vi "颗粒滤波3 filter.vi"() -> ()   [LabVIEW 2018]
uses:
  <vilib>/vision/NI_Vision_Development_Module.lvlib
panel:
  in  "Selection Values":T2(array[cluster])=[{"Measurement Parameter"=39, "Range Lower Value"=5.0, "Range Upper Value"=10000000.0, "Range"=FALSE, "Measurement Type"=FALSE}] {"Measurement Parameter" items=["Center of Mass X", "Center of Mass Y", "First Pixel X", "First Pixel Y", "Bounding Rect Left", "Bounding Rect Top", "Bounding Rect Right", "Bounding Rect Bottom", "Max Feret Diameter Start X", "Max Feret Diameter Start Y", "Max Feret Diameter End X", "Max Feret Diameter End Y", "Max Horiz. Segment Length Left", "Max Horiz. Segment Length Right", "Max Horiz. Segment Length Row", "-", "Bounding Rect Width", "Bounding Rect Height", "Bounding Rect Diagonal", "Perimeter", "Convex Hull Perimeter", "Holes' Perimeter", "Max Feret Diameter", "Equivalent Ellipse Major Axis", "Equivalent Ellipse Minor Axis", "Equivalent Ellipse Minor Axis (Feret)", "Equivalent Rect Long Side", "Equivalent Rect Short Side", "Equivalent Rect Diagonal", "Equivalent Rect Short Side (Feret)", "Average Horiz. Segment Length", "Average Vert. Segment Length", "Hydraulic Radius", "Waddel Disk Diameter", "-", "Area", "Holes' Area", "Particle & Holes' Area", "Convex Hull Area", "Image Area", "-", "Number of Holes", "Number of Horiz. Segments", "Number of Vert. Segments", "-", "Orientation", "Max Feret Diameter Orientation", "-", "% Area/Image Area", "% Area/(Particle & Holes' Area)", "Ratio of Equivalent Ellipse Axes", "Ratio of Equivalent Rect Sides", "-", "Elongation Factor", "Compactness Factor", "Heywood Circularity Factor", "Type Factor", "-", "Sum X", "Sum Y", "Sum XX", "Sum XY", "Sum YY", "Sum XXX", "Sum XXY", "Sum XYY", "Sum YYY", "-", "Moment of Inertia XX", "Moment of Inertia XY", "Moment of Inertia YY", "Moment of Inertia XXX", "Moment of Inertia XXY", "Moment of Inertia XYY", "Moment of Inertia YYY", "Norm. Moment of Inertia XX", "Norm. Moment of Inertia XY", "Norm. Moment of Inertia YY", "Norm. Moment of Inertia XXX", "Norm. Moment of Inertia XXY", "Norm. Moment of Inertia XYY", "Norm. Moment of Inertia YYY", "Hu Moment 1", "Hu Moment 2", "Hu Moment 3", "Hu Moment 4", "Hu Moment 5", "Hu Moment 6", "Hu Moment 7"]}
  in  "Tab Control":T3(tab)
  out "Original":T4(plugin-control) caption="Original Image"
  out "Threshold":T4(plugin-control) caption="Threshold Image"
  out "Fill Hole and Reject Border":T4(plugin-control) caption="Reject Border and Fill Holes"
  out "Filter and Overlay Area":T4(plugin-control) caption="Filter Out Non Circles and Overlay Particle Area"
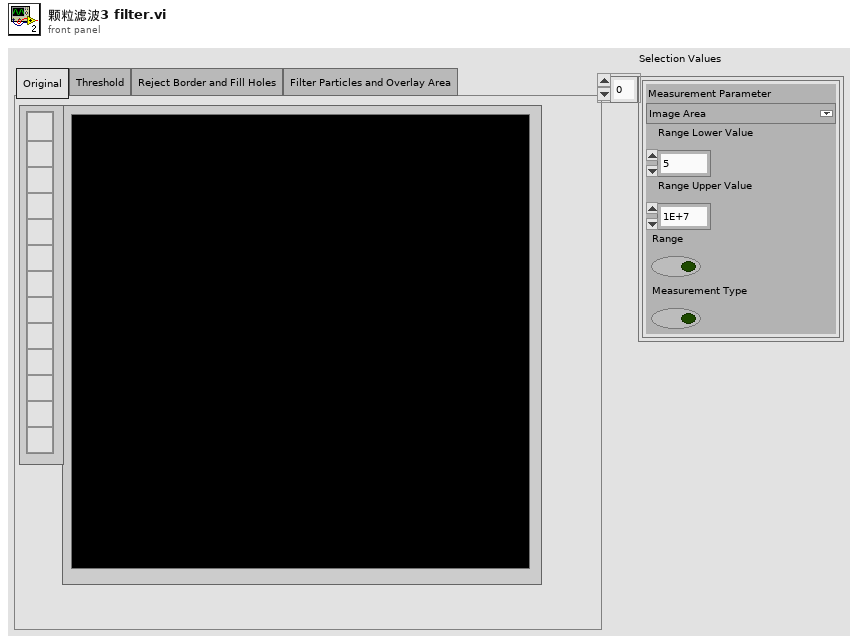
[diagram p1: front panel]
types:
  T1 = typedef "Particle Parameters" = i32
  T2 = cluster{"Measurement Parameter":T1, "Range Lower Value":dbl, "Range Upper Value":dbl, "Range":bool, "Measurement Type":bool}[]
  T3 = enum32{"Original", "Threshold", "Reject Border and Fill Holes", "Filter Particles and Overlay Area"}
  T4 = typedef "IMAQ Image.ctl" = refnum<image>
  T5 = typedef "Image Type" = u32
  T6 = cluster{"Desired Font (Application)":enum16{"User-specified Font", "Application Font", "System Font", "Dialog Font"}, "[User-specified Font]":cluster{"Font Name":string, "Size":i16, "Strikeout?":bool, "Italic?":bool, "Underline?":bool, "Outline?":bool, "Shadow?":bool, "Bold?":bool, "Rotation Angle":dbl}, "Horizontal Alignment":i16, "Vertical Alignment":i16}
  T7 = cluster{"Particle Measurements (Pixels)[0]":dbl, "Particle Measurements (Pixels)[1]":dbl, "Particle Measurements (Pixels)[2]":dbl}
  T8 = cluster{"Particle Measurements (Pixels)[0]":dbl, "Particle Measurements (Pixels)[1]":dbl}
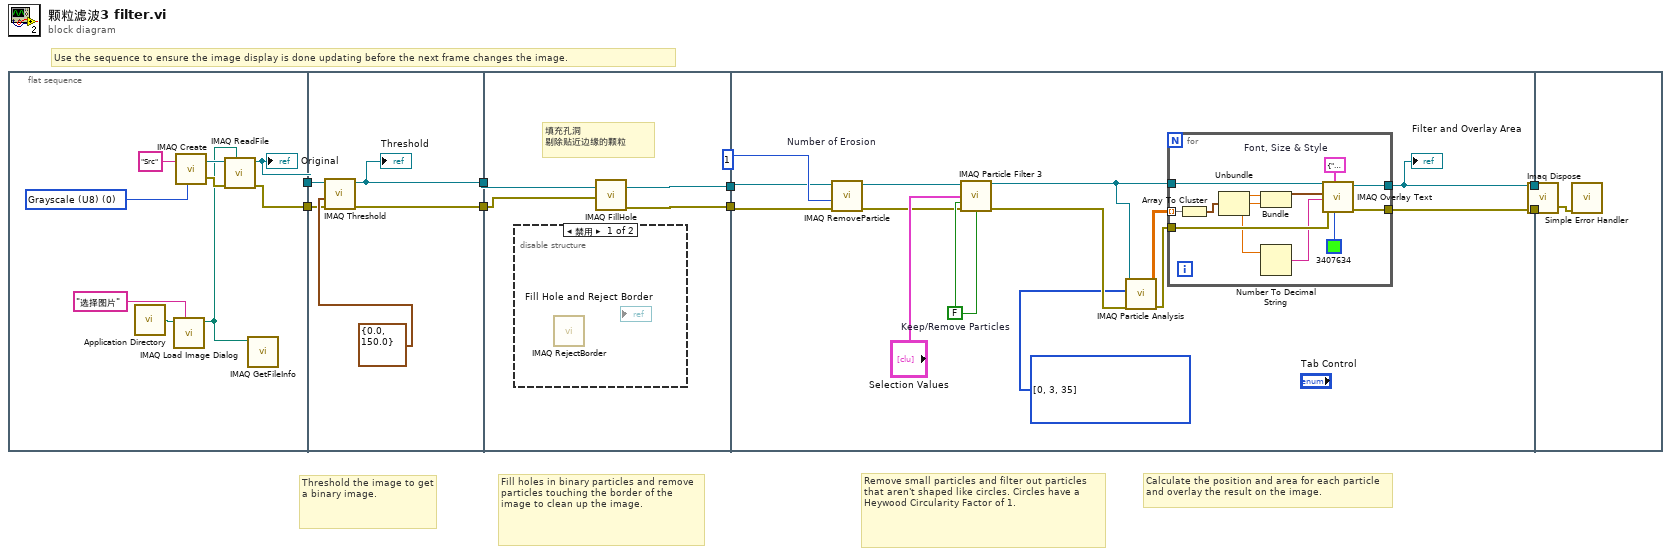
[diagram p0: block diagram]
diagram:
  # "Use the sequence to ensure the image display is done updating before the next frame changes the image."
  # "Calculate the position and area for each particle and overlay the result on the image."
  # "Remove small particles and filter out particles that aren't shaped like circles. Circles have a Heywood Circularity Factor of 1."
  # "Fill holes in binary particles and remove particles touching the border of the image to clean up the image."
  # "Threshold the image to get a binary image."
  n1 = flat-sequence {
    tunnel: [w11] -> w8
    tunnel: [w10] -> w7
    tunnel: [w20] -> w6
    tunnel: [w21] -> w5
    tunnel: w8 -> [w19]
    tunnel: w7 -> [w18]
    tunnel: w6 -> [w26]
    tunnel: w5 -> [w25]
    tunnel: [w24] -> w3
    tunnel: [w23] -> w4
    tunnel: w4 -> [w30]
    tunnel: w3 -> [w29]
    tunnel: [w36] -> w2
    tunnel: [w28] -> w1
    tunnel: w2 -> [w55]
    tunnel: w1 -> [w56]
    frame #0 {
      w12 = T5 0 items=["Grayscale (U8)", "Grayscale (I16)", "Grayscale (SGL)", "Complex (CSG)", "RGB (U32)", "HSL (U32)", "RGB (U64)", "Grayscale (U16)"] ("Image Type")
      n2 = call <vilib>:"Application Directory.vi"() -> ("Application Directory"=w13:path)
      n3 = call "IMAQ Load Image Dialog"("Prompt"="选择图片" ("prompt"), "Start Path"=w13) -> ("Path"=w9:path)  [unwired: 7 in, 2 out]
      n4 = call "IMAQ Create"("Image Name"="Src", "Image Type"=w12) -> ("New Image"=w16:T4, "error out"=w15:errorcluster)  [unwired: 3 in]
      n5 = call "IMAQ ReadFile"("File Path"=w9, "error in (no error)"=w15, "Image"=w16) -> ("error out"=w10:errorcluster, "Image Out"=w11:T4)  [unwired: 4 in, 3 out]
      "Original" <- w11
      n6 = call "IMAQ GetFileInfo"("File Path"=w9) -> ()  [unwired: 4 in, 7 out]
    }
    frame #1 {
      n7 = call "IMAQ Threshold"("error in (no error)"=w18, "Range"=cluster{"Lower value":sgl, "Upper value":sgl} {"Lower value"=0.0, "Upper value"=150.0}, "Image Src"=w19) -> ("error out"=w21:errorcluster, "Image Dst Out"=w20:T4)  [unwired: 7 in]
      "Threshold" <- w20
    }
    frame #2 {
      # "填充孔洞\n剔除贴近边缘的颗粒"
      n8 = disable-structure shown="禁用" {
        frame Disabled {
          n9 = call "IMAQ RejectBorder"() -> ()  [unwired: 6 in, 2 out]
        }
        frame Enabled {
        }
      }
      n10 = call "IMAQ FillHole"("error in (no error)"=w25, "Image Src"=w26) -> ("error out"=w23:errorcluster, "Image Dst Out"=w24:T4)  [unwired: 4 in]
    }
    frame #3 {
      w33 = 1  # Number of Erosion
      w35 = FALSE  # Keep/Remove Particles
      w37 = T1[] [0, 3, 35] items=["Center of Mass X", "Center of Mass Y", "First Pixel X", "First Pixel Y", "Bounding Rect Left", "Bounding Rect Top", "Bounding Rect Right", "Bounding Rect Bottom", "Max Feret Diameter Start X", "Max Feret Diameter Start Y", "Max Feret Diameter End X", "Max Feret Diameter End Y", "Max Horiz. Segment Length Left", "Max Horiz. Segment Length Right", "Max Horiz. Segment Length Row", "-", "Bounding Rect Width", "Bounding Rect Height", "Bounding Rect Diagonal", "Perimeter", "Convex Hull Perimeter", "Holes' Perimeter", "Max Feret Diameter", "Equivalent Ellipse Major Axis", "Equivalent Ellipse Minor Axis", "Equivalent Ellipse Minor Axis (Feret)", "Equivalent Rect Long Side", "Equivalent Rect Short Side", "Equivalent Rect Diagonal", "Equivalent Rect Short Side (Feret)", "Average Horiz. Segment Length", "Average Vert. Segment Length", "Hydraulic Radius", "Waddel Disk Diameter", "-", "Area", "Holes' Area", "Particle & Holes' Area", "Convex Hull Area", "Image Area", "-", "Number of Holes", "Number of Horiz. Segments", "Number of Vert. Segments", "-", "Orientation", "Max Feret Diameter Orientation", "-", "% Area/Image Area", "% Area/(Particle & Holes' Area)", "Ratio of Equivalent Ellipse Axes", "Ratio of Equivalent Rect Sides", "-", "Elongation Factor", "Compactness Factor", "Heywood Circularity Factor", "Type Factor", "-", "Sum X", "Sum Y", "Sum XX", "Sum XY", "Sum YY", "Sum XXX", "Sum XXY", "Sum XYY", "Sum YYY", "-", "Moment of Inertia XX", "Moment of Inertia XY", "Moment of Inertia YY", "Moment of Inertia XXX", "Moment of Inertia XXY", "Moment of Inertia XYY", "Moment of Inertia YYY", "Norm. Moment of Inertia XX", "Norm. Moment of Inertia XY", "Norm. Moment of Inertia YY", "Norm. Moment of Inertia XXX", "Norm. Moment of Inertia XXY", "Norm. Moment of Inertia XYY", "Norm. Moment of Inertia YYY", "Hu Moment 1", "Hu Moment 2", "Hu Moment 3", "Hu Moment 4", "Hu Moment 5", "Hu Moment 6", "Hu Moment 7"] ("Pixel Measurements")
      n11 = call "IMAQ RemoveParticle"("error in (no error)"=w30, "Number of Erosion"=w33, "Image Src"=w29) -> ("error out"=w31:errorcluster, "Image Dst Out"=w32:T4)  [unwired: 7 in]
      n12 = call "IMAQ Particle Filter 3"("Image Src"=w32, "Selection Values"="Selection Values", "Keep/Remove Particles (F)"=w35, "error in (no error)"=w31, "Fill Holes? (F)"=w35) -> ("Image Dst Out"=w40:T4, "error out"=w41:errorcluster)  [unwired: 8 in, 1 out]
      n13 = call "IMAQ Particle Analysis"("error in (no error)"=w41, "Pixel Measurements"=w37, "Image"=w40) -> ("error out"=w38:errorcluster, "Particle Measurements (Pixels)"=w39:dbl[][])  [unwired: 3 in, 4 out]
      n14 = for {
        tunnel: w38 -> [w54]
        tunnel: [w53] -> w36
        tunnel: [w52] -> w28
        tunnel: w40 -> [w49]
        tunnel: w39 -> [w43] mode=indexing
        w42 = T6 {"Desired Font (Application)"=enum."Application Font", "[User-specified Font]"={"Font Name"="", "Size"=12, "Strikeout?"=FALSE, "Italic?"=FALSE, "Underline?"=FALSE, "Outline?"=FALSE, "Shadow?"=FALSE, "Bold?"=FALSE, "Rotation Angle"=0.0}, "Horizontal Alignment"=0, "Vertical Alignment"=0}  # Font, Size & Style
        n15 = Array To Cluster(array=w43) -> (cluster=w48:T7)
        n16 = Unbundle(w48) -> ("Particle Measurements (Pixels)[0]"=w47:dbl, "Particle Measurements (Pixels)[1]"=w46:dbl, "Particle Measurements (Pixels)[2]"=w44:dbl)
        n17 = Bundle("Particle Measurements (Pixels)[0]"=w47, "Particle Measurements (Pixels)[1]"=w46) -> (w45:T8)  [unwired: 1 in]
        n18 = Number To Decimal String(number=w44) -> (decimal integer string=w51:string)  [unwired: 1 in]
        n19 = call "IMAQ Overlay Text"("Text Color (black)"=u32 3407634, "Font, Size & Style"=w42, "error in (no error)"=w54, "String"=w51, "Origin"=w45, "Image"=w49) -> ("error out"=w53:errorcluster, "Image Out"=w52:T4)  [unwired: 4 in]
      }
      "Filter and Overlay Area" <- w28
    }
    frame #4 {
      n20 = call "Imaq Dispose"("Image"=w56, "error in (no error)"=w55) -> ("error out"=w57:errorcluster)  [unwired: 4 in]
      n21 = call <vilib>:"Simple Error Handler.vi"("error in (no error)"=w57) -> ()  [unwired: 4 in, 5 out]
    }
  }
